vi "UsrProfiles-Select new user.vi"(9 "New user name":string) -> ()   [LabVIEW 2020]
uses:
  Typedefs/Save-Load enum.ctl
  Globals/gl_UsrProfiles globals.vi
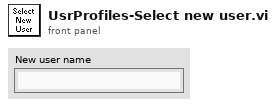
[diagram p1: front panel]
types:
  T1 = typedef "Save-Load enum.ctl" = enum16{"Save to file", "Load from file", "Compare from file", "Save Backup"}
  T2 = typedef "User login window refs.ctl" = cluster{"User profiles window ref":refnum<k9>, "Users listbox":refnum<vi>, "Profiles listbox":refnum<vi>, "Last used":refnum<vi>}
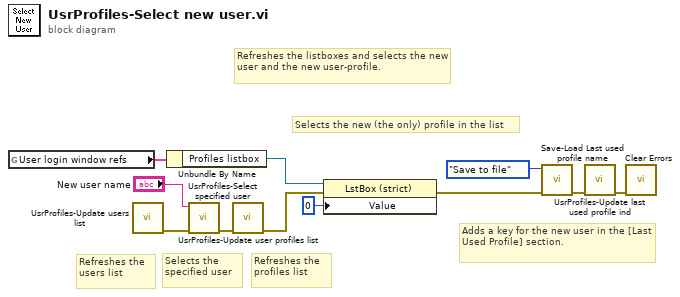
[diagram p0: block diagram]
diagram:
  # "Adds a key for the new user in the [Last Used Profile] section."
  # "Selects the specified user"
  # "Refreshes the profiles list"
  # "Selects the new (the only) profile in the list"
  # "Refreshes the users list"
  # "Refreshes the listboxes and selects the new user and the new user-profile."
  n1 = global read "gl_UsrProfiles globals.vi" "User login window refs"() -> (w5:T2)
  n2 = call "UsrProfiles-Update users list.vi"() -> ("error out"=w9:errorcluster)  [unwired: 10 in, 1 out]
  n3 = Unbundle By Name(w5) -> ("Profiles listbox"=w10:refnum<vi>)
  n4 = call "UsrProfiles-Select specified user.vi"("error in (no error)"=w9, "New user name"="New user name") -> ("error out"=w8:errorcluster)  [unwired: 9 in]
  n5 = call "UsrProfiles-Update user profiles list.vi"("error in"=w8) -> ("error out"=w6:errorcluster)  [unwired: 9 in, 1 out]
  n6 = property on="Property Node" class="LstBox (strict)"(reference=w10, error in=w6, "Value"=0) -> (error out=w3:errorcluster)  [unwired: 1 out]
  n7 = call "Save-Load Last used profile name.vi"("error in"=w3, "Function"=Save-Load_enum."Save to file") -> ("error out"=w2:errorcluster)  [unwired: 7 in, 2 out]
  n8 = call "UsrProfiles-Update last used profile ind.vi"("error in"=w2) -> ("error out"=w1:errorcluster)  [unwired: 10 in]
  n9 = call <vilib>:"Clear Errors.vi"("error in (no error)"=w1) -> ()  [unwired: 5 in, 2 out]
